vi "sv_Get LabVIEW Datatype String.vi"(4 "LabVIEW datatype":T1 items=["String: abc"=7, "Boolean: True or False"=8, "Scalar: y"=0, "Array: Y"=1, "Waveform: t0, dt, Y, variant"=2, "Cluster: x0, dx, Y"=3, "Cluster: X, Y"=4, "Waterfall"=5, "Colormap"=6]) -> (1 "datatype string":string)   [LabVIEW 2017]
uses:
  <vilib>/addons/_NISVFA/_Shared subVIs/Controls/LV Datatypes.ctl
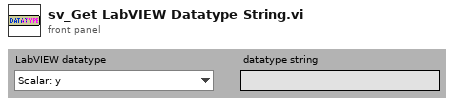
[diagram p1: front panel]
types:
  T1 = typedef "LV Datatypes.ctl" = i32
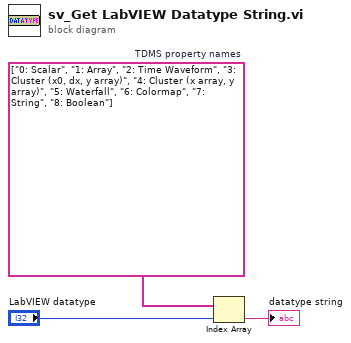
[diagram p0: block diagram]
diagram:
  w1 = string[] ["0: Scalar", "1: Array", "2: Time Waveform", "3: Cluster (x0, dx, y array)", "4: Cluster (x array, y array)", "5: Waterfall", "6: Colormap", "7: String", "8: Boolean"]  # TDMS property names
  n1 = Index Array(array=w1, index="LabVIEW datatype") -> (element=→"datatype string":string)
